vi "Is State Visible.vi"(11 "Visibility":T1) -> (3 "Visible":bool)   [LabVIEW 2020, in "OOPanel.lvlib" / "Panel.lvclass"]
uses:
  Panel.lvclass
  Visibility State.ctl
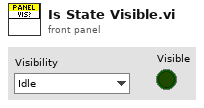
[diagram p1: front panel]
types:
  T1 = typedef "OOPanel.lvlib/Panel.lvclass/Visibility State.ctl" = enum16{"Idle", "Closed", "Hidden", "Visible", "Subpanel"}
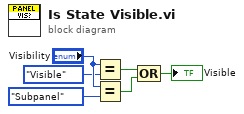
[diagram p0: block diagram]
diagram:
  n1 = Equal?(x="Visibility", y=Visibility_State."Visible") -> (x = y?=w3:bool)
  n2 = Equal?(x="Visibility", y=Visibility_State."Subpanel") -> (x = y?=w2:bool)
  n3 = Compound Arithmetic op=OR(w3, w2) -> (→"Visible":bool)
